vi "Array splitten.vi"(8 "error in (no error)":errorcluster caption="Fehler (Eingang, kein Fehler)", 11 "Array":dbl[](array[numeric])) -> (0 "error out":errorcluster caption="Fehler (Ausgang)", 1 "Ungerader Index":dbl[](array[numeric]), 3 "Gerader Index":dbl[](array[numeric]))   [LabVIEW 2020, in "EPA 1065.lvlib" / "T90 Test 1065-308.lvlib"]
uses:
  T90 Test 1065-308.lvlib
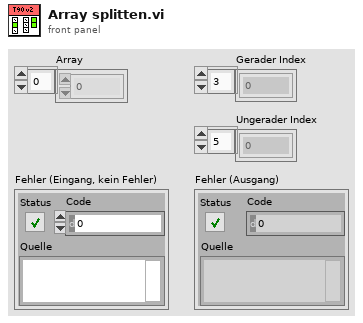
[diagram p1: front panel]
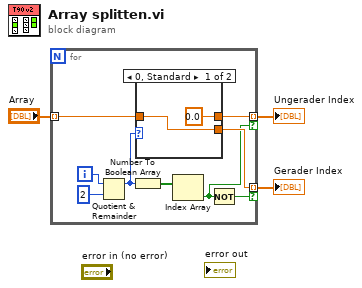
[diagram p0: block diagram]
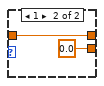
[diagram p2: hidden frame]
diagram:
  n1 = for {
    tunnel: "Array" -> [w10] mode=indexing
    tunnel: [w9] -> w3 mode=indexing if=w5
    tunnel: [w8] -> w2 mode=indexing if=w4
    i -> [w12]
    n2 = Quotient & Remainder(x=w12, y=2) -> (x-y*floor(x/y)=w7:i32)  [unwired: 1 out]
    n3 = Number To Boolean Array(number=w7) -> (Boolean array=w6:bool[])
    n4 = case shown="0, Standard" w7 {
      tunnel: w10 -> [w14 w16]
      tunnel: [w14 0.0 ("seconds since 1Jan1904")] -> w9
      tunnel: [0.0 ("seconds since 1Jan1904") w16] -> w8
      frame 0, Default {
      }
      frame 1 {
      }
    }
    n5 = Index Array(array=w6) -> (element=w4:bool)  [unwired: 1 in]
    n6 = Not(x=w4) -> (.not. x?=w5:bool)
  }
  "Gerader Index" <- w3
  "Ungerader Index" <- w2
